vi "Read IFD.vi"(8 "error in":errorcluster, 9 "IFDOffset":u32, 10 "Tiff Bitness":T1(ring), 11 "Byte Stream File in":refnum<file>) -> (0 "error out":errorcluster, 1 "NextIDOOffset":u32, 2 "Array":T3(array[cluster]), 3 "refnum out":refnum<file>)   [LabVIEW 2020, in "LV Tiff.lvlib"]
uses:
  LV Tiff.lvlib
  Tiff Data Type.ctl
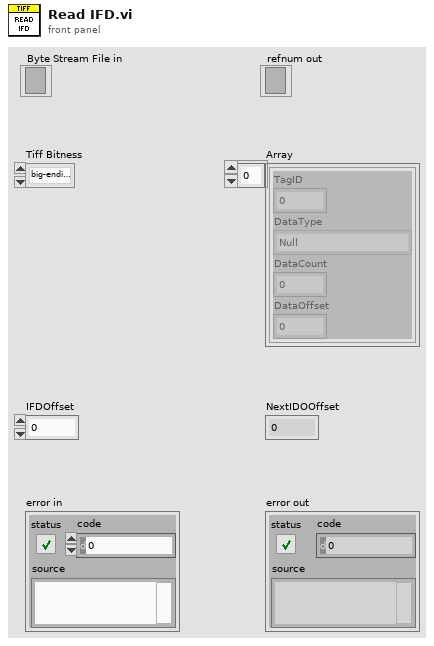
[diagram p1: front panel]
types:
  T1 = enum16{"big-endian, network order", "native, host order", "little-endian"}
  T2 = typedef "LV Tiff.lvlib/Tiff Data Type.ctl" = enum16{"Null", "BYTE", "ASCII", "SHORT", "LONG", "RATIONAL", "SBYTE", "UNDEFINE", "SSHORT", "SLONG", "SRATIONAL", "FLOAT", "DOUBLE"}
  T3 = cluster{"TagID":u16, "DataType":T2, "DataCount":u32, "DataOffset":u32}[]
  T4 = cluster{"TagID":u16, "DataType":T2, "DataCount":u32, "DataOffset":u32}
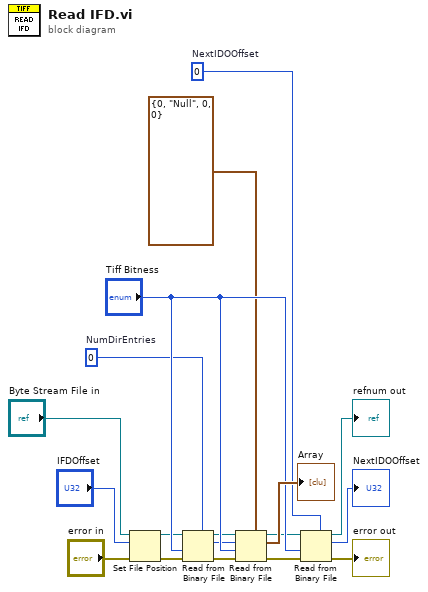
[diagram p0: block diagram]
diagram:
  w16 = u32 0  # NextIDOOffset
  w7 = u16 0  # NumDirEntries
  n1 = Set File Position(offset (in bytes) (0)="IFDOffset", refnum="Byte Stream File in", error in="error in") -> (refnum out=w9:refnum<file>, error out=w4:errorcluster)  [unwired: 1 in]
  n2 = Read from Binary File(5:w7, 8:w4, 9:"Tiff Bitness", 11:w9) -> (0:w3:errorcluster, 2:w12:u16, 3:w13:refnum<file>)  [unwired: 2 in, 1 out]
  n3 = Read from Binary File(5:T4 {"TagID"=0, "DataType"=enum."Null", "DataCount"=0, "DataOffset"=0}, 8:w3, 9:"Tiff Bitness", 10:w12, 11:w13) -> (0:w2:errorcluster, 2:→"Array":T3, 3:w14:refnum<file>)  [unwired: 1 in, 1 out]
  n4 = Read from Binary File(5:w16, 8:w2, 9:"Tiff Bitness", 11:w14) -> (0:→"error out":errorcluster, 2:→"NextIDOOffset":u32, 3:→"refnum out":refnum<file>)  [unwired: 2 in, 1 out]
